vi "Graph Element.vi"() -> ()   [LabVIEW 2013]
panel:
  in  "PointStyle":u16(ring) caption="0"
  in  "Interpolation":u16(ring) caption="2"
  in  "LineWidth":u16(ring) caption="0"
  in  "LineStyle":u16(ring) caption="0"
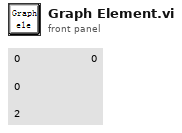
[diagram p1: front panel]
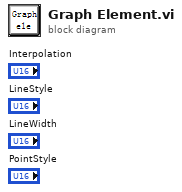
[diagram p0: block diagram]
diagram:
